vi "place lines.vi"(7 "picture in":picture, 9 "line":u16(ring) items=["kalpha", "kbeta", "lalpha", "lbeta", "escape", "sum"], 10 "Graph":refnum<vi>, 11 "Energy":dbl format="%#_13g") -> (3 "line to place":picture)   [LabVIEW 2023]
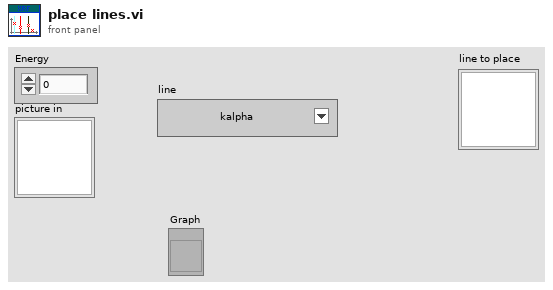
[diagram p1: front panel]
types:
  T1 = cluster{"Width":u16, "Style":enum32{"Solid", "Dash", "Dot", "DashDot", "DashDotDot"}}
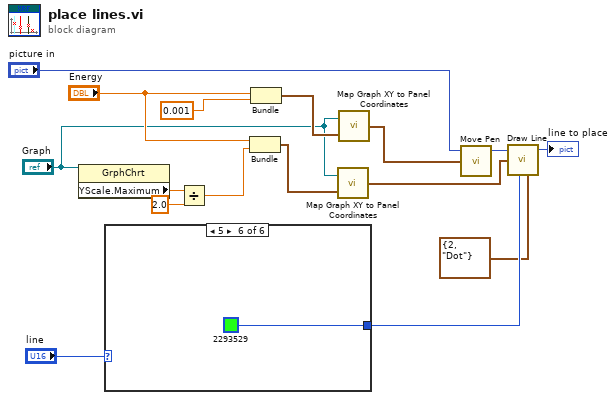
[diagram p0: block diagram]
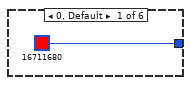
[diagram p2: hidden frame]
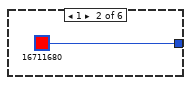
[diagram p3: hidden frame]
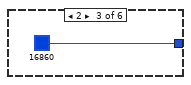
[diagram p4: hidden frame]
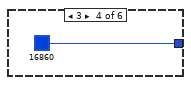
[diagram p5: hidden frame]
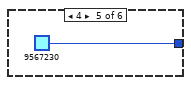
[diagram p6: hidden frame]
diagram:
  n1 = property class="GrphChrt"(reference="Graph") -> ("YScale.Maximum"=w16:dbl)  [unwired: 1 in, 2 out]
  n2 = case shown="5" "line" {
    tunnel: [u32 16711680 u32 16711680 u32 16860 u32 16860 u32 9567230 u32 2293529] -> w8
    frame 0, Default {
    }
    frame 1 {
    }
    frame 2 {
    }
    frame 3 {
    }
    frame 4 {
    }
    frame 5 {
    }
  }
  n3 = Divide(x=w16, y=2.0) -> (x/y=w14:dbl)
  n4 = Bundle("Energy"="Energy", w14) -> (w5:cluster{"Energy":dbl, dbl})  [unwired: 1 in]
  n5 = Bundle("Energy"="Energy", "y"=0.001) -> (w3:cluster{"Energy":dbl, "y":dbl})  [unwired: 1 in]
  n6 = call "Map Graph XY to Panel Coordinates.vi"("XY"=w5, "Graph"="Graph") -> ("Coords"=w4:cluster{i32, i32})
  n7 = call "Map Graph XY to Panel Coordinates.vi"("XY"=w3, "Graph"="Graph") -> ("Coords"=w2:cluster{i32, i32})
  n8 = call <vilib>:"Move Pen.vi"("new position"=w2, "picture"="picture in") -> ("new picture"=w10:picture)  [unwired: 3 in]
  n9 = call <vilib>:"Draw Line.vi"("picture"=w10, "end point"=w4, "color(black)"=w8, "pen"=T1 {"Width"=2, "Style"=enum."Dot"}) -> ("new picture"=→"line to place":picture)  [unwired: 5 in]
